vi "Page - Ports.vi"(8 "error in (no error)":errorcluster, 11 "Node Ptr":T3 format="%.0x") -> (0 "error out":errorcluster)   [LabVIEW 2020, in "SLSC-12201 DIO System Explorer.lvlib"]
uses:
  SLSC-12201 DIO System Explorer.lvlib
  <vilib>/NI VeriStand/Custom Device API/Custom Device API.lvlib
  <vilib>/NI VeriStand/Custom Device API/Custom Device Item Ref.ctl
  <vilib>/Utility/miscctls.llb/LVRowAndColumnTypeDef.ctl
  Direction Control.ctl
panel:
  in  "Apply":bool
  in  "Port Type":T1 items=["Input", "Output Source", "Output Sink", "Output Push-Pull"]
  out "Cell Position":T2
  in  "Type":u16(ring) items=["Input", "Output Source", "Output Sink", "Output Pull-up"]
  out "Multicolumn Listbox":i32(listbox)=4
  in  "Disable Port":bool
  in  "Enable Port":bool
  in  "SHDocVw.IWebBrowser2":refnum<k7>(container)
  in  "Header":cluster{"Section Name":string}={"Section Name"="Custom Device Item Settings"}
  in  "Description":string
  out "Name":string
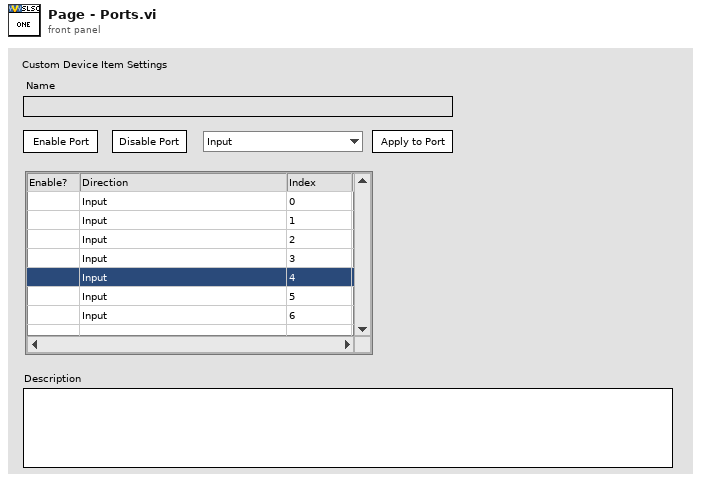
[diagram p1: front panel]
types:
  T1 = typedef "SLSC-12201 DIO System Explorer.lvlib/Direction Control.ctl" = u16
  T2 = typedef "LVRowAndColumnTypeDef.ctl" = cluster{"Row":i32, "Column":i32}
  T3 = typedef "Custom Device API.lvlib/Custom Device Item Ref.ctl" = u64
  T4 = typedef "Custom Device API.lvlib/Custom Device Item Info.ctl" = cluster{"Name":string, "Is Channel":bool, "GUID":string, "Is Waveform":bool}
  T5 = typedef "Custom Device API.lvlib/Custom Device Channel.ctl" = cluster{"Type":T6, "Units":string, "Default Value":dbl, "Faultable":bool, "Scalable":bool}
  T6 = typedef "Custom Device API.lvlib/Custom Device Channel Type.ctl" = enum16{"Input", "Output"}
  T7 = cluster{"Channel Name":string, "SLSC Name":string, "Channel":T5, "Enum Names":string[], "Enum Values":i32[]}[]
  T8 = typedef "Custom Device API.lvlib/Custom Device Commands.ctl" = enum16{"Default", "Item renamed", "Shutdown", "Dynamic button pressed"}
  T9 = typedef "LVPoint32TypeDef.ctl" = cluster{"Horizontal":i32, "Vertical":i32}
  T10 = typedef "LVPositionTypeDef.ctl" = cluster{"Left":i32, "Top":i32}
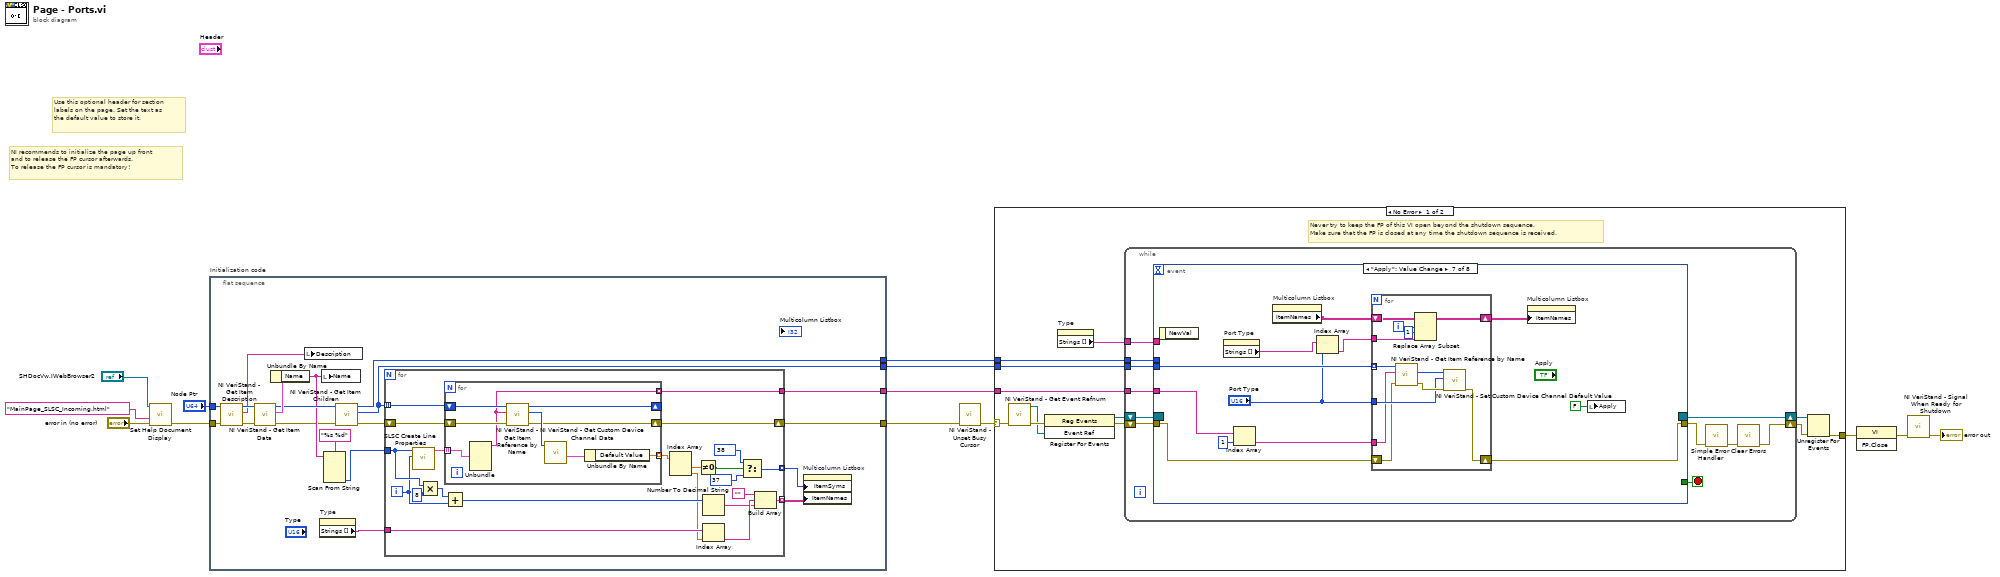
[diagram p0: block diagram]
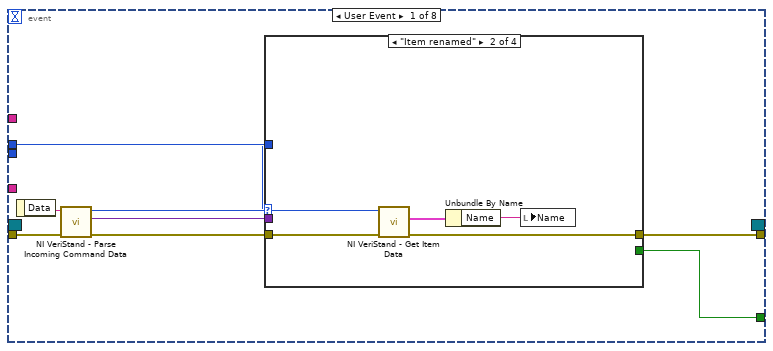
[diagram p2: hidden frame]
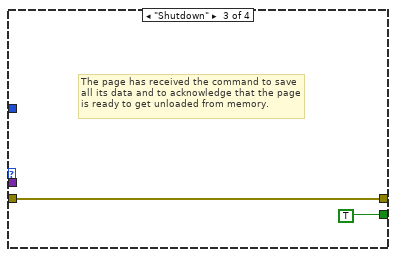
[diagram p4: hidden frame]
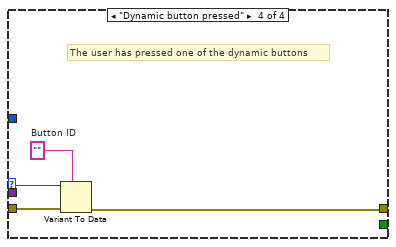
[diagram p5: hidden frame]
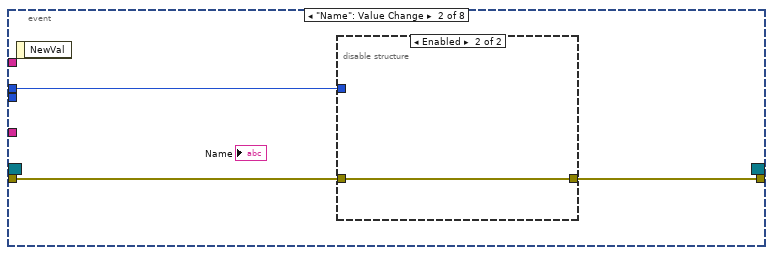
[diagram p6: hidden frame]
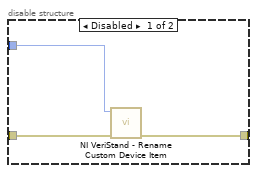
[diagram p7: hidden frame]
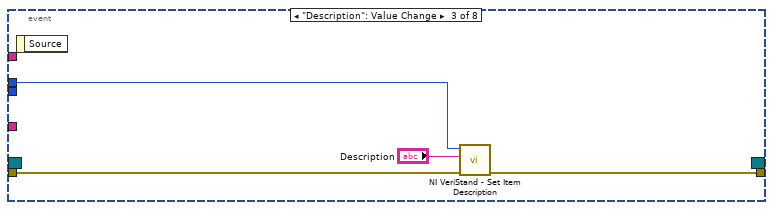
[diagram p8: hidden frame]
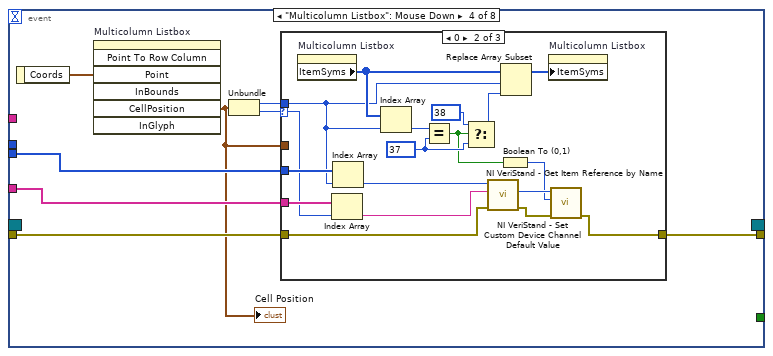
[diagram p9: hidden frame]
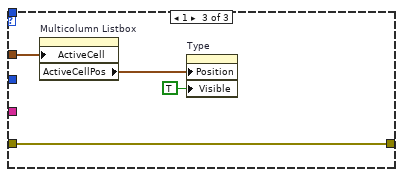
[diagram p11: hidden frame]
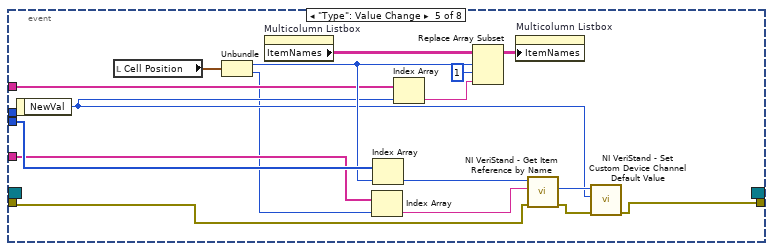
[diagram p12: hidden frame]
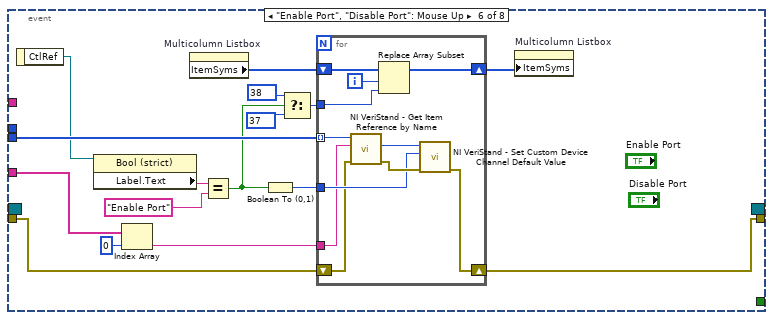
[diagram p13: hidden frame]
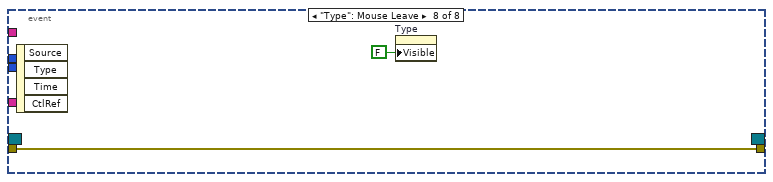
[diagram p14: hidden frame]
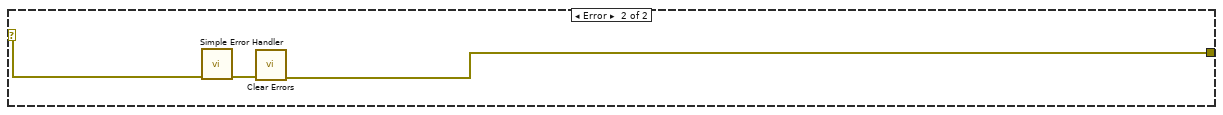
[diagram p15: hidden frame]
diagram:
  # "Use this optional header for section labels on the page. Set the text as the default value to store it."
  # "NI recommends to initialize the page up front\nand to release the FP cursor afterwards.\nTo release the FP cursor is mandatory!"
  n1 = call "Set Help Document Display.vi"("error in (no error)"="error in (no error)", "HTML File to Load"="MainPage_SLSC_Incoming.html" ("HTML File"), "SHDocVw.IWebBrowser2"="SHDocVw.IWebBrowser2") -> ("error out"=w3:errorcluster)  [unwired: 8 in]
  n2 = flat-sequence "Initialization code" {
    tunnel: w3 -> [w31]
    tunnel: "Node Ptr" -> [w30]
    tunnel: [w26] -> w9
    tunnel: [w24] -> w7
    tunnel: [w20] -> w2
    tunnel: [w19] -> w1
    frame #0 {
      n3 = call <vilib>:"NI VeriStand - Get Item Description.vi"("error in (no error)"=w31, "Item Ref in"=w30) -> ("error out"=w28:errorcluster, "Description"=w29:string, "Item Ref out"=w32:T3)  [unwired: 7 out]
      n4 = call <vilib>:"NI VeriStand - Get Item Data.vi"("error in (no error)"=w28, "Item Ref in"=w32) -> ("error out"=w18:errorcluster, "Item Info"=w27:T4, "Item Ref out"=w25:T3)  [unwired: 7 out]
      n5 = Unbundle By Name(w27) -> ("Name"=w22:string)
      n6 = local write "Description"(w29) -> ()
      n7 = property on="Type" class="Ring (strict)"() -> ("Strings []"=w16:string[])  [unwired: 2 in, 2 out]
      n8 = local write "Name"(w22) -> ()
      n9 = Scan From String(format string="%s %d", input string=w22) -> (output 2=w21:i32)  [unwired: 5 in, 3 out]
      n10 = call <vilib>:"NI VeriStand - Get Item Children.vi"("error in (no error)"=w18, "Item Ref in"=w25) -> ("error out"=w17:errorcluster, "Child Refs"=w20:T3[], "Item Ref out"=w24:T3)  [unwired: 6 in, 1 out]
      n11 = for {
        shift-right: [w53] -> w26
        shift-left: w17 -> [w54]
        tunnel: w20 -> [w50] mode=indexing
        tunnel: w21 -> [w47]
        tunnel: [w48] -> w19
        tunnel: w16 -> [w42]
        tunnel: [w37] -> w15 mode=indexing
        tunnel: [w33] -> w14 mode=indexing
        i -> [w44]
        n12 = call "SLSC Create Line Properties.vi"("Line Number"=w44, "Port Number"=w47) -> ("Outgoing configuration"=w52:T7)  [unwired: 9 in]
        n13 = Multiply(x=w47, y=8) -> (x*y=w45:i32)
        n14 = for {
          shift-right: [w60] -> w53
          shift-left: w54 -> [w61]
          shift-right: [w58] -> _
          shift-left: w50 -> [w59]
          tunnel: w52 -> [w57] mode=indexing
          tunnel: [w56] -> w51 mode=indexing
          tunnel: [w55] -> w48 mode=indexing
          n15 = Unbundle(w57) -> ("Channel Name"=w55:string)  [unwired: 4 out]
          n16 = call <vilib>:"NI VeriStand - Get Item Reference by Name.vi"("error in (no error)"=w61, "Item Name"=w55, "Parent Ref in"=w59) -> ("error out"=w60:errorcluster, "Item Ref"=w63:T3, "Parent Ref out"=w58:T3)  [unwired: 5 in, 1 out]
          n17 = call <vilib>:"NI VeriStand - Get Custom Device Channel Data.vi"("Channel Ref in"=w63) -> ("Channel"=w62:T5)  [unwired: 5 in, 5 out]
          n18 = Unbundle By Name(w62) -> ("Default Value"=w56:dbl)
        }
        n19 = Add(x=w45, y=w44) -> (x+y=w43:i32)
        n20 = Index Array(array=w51) -> (element #1=w49:dbl, element #2=w41:dbl)  [unwired: 2 in]
        n21 = Not Equal To 0?(x=w49) -> (x != 0?=w38:bool)
        n22 = Number To Decimal String(number=w43) -> (decimal integer string=w34:string)  [unwired: 1 in]
        n23 = Index Array(array=w42, index=w41) -> (element=w35:string)
        n24 = Select(t=38, s=w38, f=37) -> (s? t:f=w37:i32)
        n25 = Build Array("", w35, w34) -> (w33:string[])
      }
      n26 = property on="Multicolumn Listbox" class="MCListbox (strict)"("ItemSyms"=w15, "ItemNames"=w14) -> ()  [unwired: 2 in, 2 out]
    }
  }
  n27 = call <vilib>:"NI VeriStand - Unset Busy Cursor.vi"("error in (no error)"=w9) -> ("error out"=w8:errorcluster)  [unwired: 10 out]
  n28 = case shown="No Error" w8 {
    selector: w8 -> [w67 w221]
    tunnel: [w72 w219] -> w13
    tunnel: w7 -> [w68 _]
    tunnel: w2 -> [w66 _]
    tunnel: w1 -> [w65 _]
    frame No Error {
      # "Never try to keep the FP of this VI open beyond the shutdown sequence.\nMake sure that the FP is closed at any time the shutdown sequence is received."
      n29 = call <vilib>:"NI VeriStand - Get Event Refnum.vi"("error in (no error)"=w67) -> ("error out"=w75:errorcluster, "Event Ref"=w71:refnum<user-event>)  [unwired: 9 out]
      n30 = register-events(error in=w75, w71) -> (reference out=w69:refnum<event-registration>, error out=w70:errorcluster)  [unwired: 1 in]
      n31 = property on="Type" class="Ring (strict)"() -> ("Strings []"=w64:string[])  [unwired: 2 in, 2 out]
      n32 = while {
        tunnel: w68 -> [w82]
        shift-right: [w79] -> w73
        shift-left: w70 -> [w85]
        shift-right: [w86] -> w74
        shift-left: w69 -> [w84]
        tunnel: w66 -> [w78]
        tunnel: w65 -> [w77]
        tunnel: w64 -> [w76]
        stop <- w83 stop-if-true
        n33 = event shown="[6] \"Apply\": Value Change" {
          selector: w84 -> [_ _ _ _ _ _ _ _]
          dyn-events: [_ _ _ _ _ _ _ _] -> w86
          timeout: _ -> [_ _ _ _ _ _ _ _]
          tunnel: w85 -> [w94 w109 w116 w120 w152 w171 w200 w218]
          tunnel: [w90 _ _ _ _ _ _ _] -> w83
          tunnel: [w89 w108 w115 w119 w150 w170 w199 w218] -> w81
          tunnel: w82 -> [w88 w107 w117 _ _ _ _ _]
          tunnel: w78 -> [_ _ _ w122 w156 w181 w204 _]
          tunnel: w77 -> [_ _ _ w121 w155 w174 w203 _]
          tunnel: w76 -> [_ _ _ _ w151 _ _ _]
          event User Event {
            n34 = event-data() -> ("Data"=w93:string)  [unwired: 1 out]
            n35 = call <vilib>:"NI VeriStand - Parse Incoming Command Data.vi"("error in (no error)"=w94, "Incoming data"=w93) -> ("error out"=w92:errorcluster, "Outgoing data"=w87:variant, "Action"=w91:T8)  [unwired: 7 out]
            n36 = case shown="\"Item renamed\"" w91 {
              tunnel: w92 -> [w95 w100 w101 w106]
              tunnel: [_ _ TRUE _] -> w90
              tunnel: [w95 w97 w101 w103] -> w89
              tunnel: w88 -> [_ w99 _ _]
              tunnel: w87 -> [_ _ _ w105]
              frame "Default", Default {
              }
              frame "Item renamed" {
                n37 = call <vilib>:"NI VeriStand - Get Item Data.vi"("error in (no error)"=w100, "Item Ref in"=w99) -> ("error out"=w97:errorcluster, "Item Info"=w98:T4)  [unwired: 8 out]
                n38 = Unbundle By Name(w98) -> ("Name"=w96:string)
                n39 = local write "Name"(w96) -> ()
              }
              frame "Shutdown" {
                # "The page has received the command to save all its data and to acknowledge that the page is ready to get unloaded from memory."
              }
              frame "Dynamic button pressed" {
                w104 = ""  # Button ID
                # "The user has pressed one of the dynamic buttons"
                n40 = Variant To Data(error in=w106, type=w104, Variant=w105) -> (error out=w103:errorcluster)  [unwired: 1 out]
              }
            }
          }
          event "Name": Value Change {
            n41 = event-data() -> ()  [unwired: 2 out]
            n42 = disable-structure shown="Enabled" {
              disable-tunnel: w109 -> [w112 w113]
              disable-tunnel: [w111 w113] -> w108
              disable-tunnel: w107 -> [w110 _]
              frame Disabled {
                n43 = call <vilib>:"NI VeriStand - Rename Custom Device Item.vi"("error in (no error)"=w112, "Item Ref in"=w110) -> ("error out"=w111:errorcluster)  [unwired: 2 in, 7 out]
              }
              frame Enabled {
              }
            }
          }
          event "Description": Value Change {
            n44 = event-data() -> ()  [unwired: 2 out]
            n45 = call <vilib>:"NI VeriStand - Set Item Description.vi"("error in (no error)"=w116, "Description"="Description", "Item Ref in"=w117) -> ("error out"=w115:errorcluster)  [unwired: 8 out]
          }
          event "Multicolumn Listbox": Mouse Down {
            n46 = event-data() -> ("Coords"=w125:T9)  [unwired: 1 out]
            n47 = invoke on="Multicolumn Listbox" class="MCListbox (strict)" method="Point To Row Column"("Point"=w125) -> ("CellPosition"=w118:T2)  [unwired: 6 in, 6 out]
            "Cell Position" <- w118
            n48 = Unbundle(w118) -> ("Row"=w123:i32, "Column"=w124:i32)
            n49 = case shown="0" w124 {
              selector: w124 -> [_ w127 _]
              tunnel: w123 -> [_ w133 _]
              tunnel: w122 -> [_ w138 _]
              tunnel: w121 -> [_ w134 _]
              tunnel: w120 -> [w126 w129 w145]
              tunnel: [w126 w128 w145] -> w119
              tunnel: w118 -> [_ _ w148]
              frame 2, Default {
              }
              frame 0 {
                w143 = 37
                n50 = property on="Multicolumn Listbox" class="MCListbox (strict)"() -> ("ItemSyms"=w140:i32[])  [unwired: 2 in, 2 out]
                n51 = Index Array(array=w134, index=w127) -> (element=w132:string)
                n52 = Index Array(array=w138, index=w133) -> (element=w135:T3)
                n53 = Index Array(array=w140, index=w133) -> (element=w142:i32)
                n54 = Equal?(x=w142, y=w143) -> (x = y?=w131:bool)
                n55 = Select(t=38, s=w131, f=w143) -> (s? t:f=w141:i32)
                n56 = call <vilib>:"NI VeriStand - Get Item Reference by Name.vi"("error in (no error)"=w129, "Item Name"=w132, "Parent Ref in"=w135) -> ("error out"=w137:errorcluster, "Item Ref"=w136:T3)  [unwired: 5 in, 2 out]
                n57 = Boolean To (0,1)(Boolean=w131) -> (0, 1=w130:i16)
                n58 = Replace Array Subset(array=w140, new element=w141, index=w133) -> (w139:i32[])
                n59 = property on="Multicolumn Listbox" class="MCListbox (strict)"("ItemSyms"=w139) -> ()  [unwired: 2 in, 2 out]
                n60 = call <vilib>:"NI VeriStand - Set Custom Device Channel Default Value.vi"("error in (no error)"=w137, "Default Value"=w130, "Channel Ref in"=w136) -> ("error out"=w128:errorcluster)  [unwired: 7 in, 1 out]
              }
              frame 1 {
                n61 = property on="Multicolumn Listbox" class="MCListbox (strict)"("ActiveCell"=w148) -> ("ActiveCellPos"=w147:T10)  [unwired: 2 in, 2 out]
                n62 = property on="Type" class="Ring (strict)"("Position"=w147, "Visible"=TRUE) -> ()  [unwired: 2 in, 2 out]
              }
            }
          }
          event "Type": Value Change {
            n63 = event-data() -> ("NewVal"=w153:u16)  [unwired: 1 out]
            n64 = local read "Cell Position"() -> (w162:T2)
            n65 = Unbundle(w162) -> ("Row"=w154:i32, "Column"=w149:i32)
            n66 = property on="Multicolumn Listbox" class="MCListbox (strict)"() -> ("ItemNames"=w165:string[][])  [unwired: 2 in, 2 out]
            n67 = Index Array(array=w155, index=w149) -> (element=w157:string)
            n68 = Index Array(array=w156, index=w154) -> (element=w158:T3)
            n69 = Index Array(array=w151, index=w153) -> (element=w161:string)
            n70 = Replace Array Subset(array=w165, new element=w161, index (row)=w154, index (col)=1 ("disabled index (col)")) -> (w164:string[][])
            n71 = property on="Multicolumn Listbox" class="MCListbox (strict)"("ItemNames"=w164) -> ()  [unwired: 2 in, 2 out]
            n72 = call <vilib>:"NI VeriStand - Get Item Reference by Name.vi"("error in (no error)"=w152, "Item Name"=w157, "Parent Ref in"=w158) -> ("error out"=w160:errorcluster, "Item Ref"=w159:T3)  [unwired: 5 in, 2 out]
            n73 = call <vilib>:"NI VeriStand - Set Custom Device Channel Default Value.vi"("error in (no error)"=w160, "Default Value"=w153, "Channel Ref in"=w159) -> ("error out"=w150:errorcluster)  [unwired: 7 in, 1 out]
          }
          event "Enable Port", "Disable Port": Mouse Up {
            n74 = event-data() -> ("CtlRef"=w178:refnum<vi>)  [unwired: 1 out]
            n75 = property class="Bool (strict)"(reference=w178) -> ("Label.Text"=w177:string)  [unwired: 1 in, 2 out]
            n76 = Index Array(array=w174, index=0) -> (element=w172:string)
            n77 = property on="Multicolumn Listbox" class="MCListbox (strict)"() -> ("ItemSyms"=w180:i32[])  [unwired: 2 in, 2 out]
            n78 = Equal?(x=w177, y="Enable Port") -> (x = y?=w169:bool)
            n79 = Boolean To (0,1)(Boolean=w169) -> (0, 1=w175:i16)
            n80 = Select(t=38, s=w169, f=37) -> (s? t:f=w166:i32)
            n81 = for {
              tunnel: w181 -> [w190] mode=indexing
              shift-right: [w187] -> w179
              shift-left: w180 -> [w188]
              tunnel: w175 -> [w186]
              tunnel: w172 -> [w185]
              shift-right: [w183] -> w170
              shift-left: w171 -> [w184]
              tunnel: w166 -> [w182]
              i -> [w189]
              n82 = call <vilib>:"NI VeriStand - Get Item Reference by Name.vi"("error in (no error)"=w184, "Item Name"=w185, "Parent Ref in"=w190) -> ("error out"=w192:errorcluster, "Item Ref"=w191:T3)  [unwired: 5 in, 2 out]
              n83 = Replace Array Subset(array=w188, new element=w182, index=w189) -> (w187:i32[])
              n84 = call <vilib>:"NI VeriStand - Set Custom Device Channel Default Value.vi"("error in (no error)"=w192, "Default Value"=w186, "Channel Ref in"=w191) -> ("error out"=w183:errorcluster)  [unwired: 7 in, 1 out]
            }
            n85 = property on="Multicolumn Listbox" class="MCListbox (strict)"("ItemSyms"=w179) -> ()  [unwired: 2 in, 2 out]
          }
          event "Apply": Value Change {
            n86 = event-data() -> ()  [unwired: 2 out]
            n87 = property on="Port Type" class="Ring (strict)"() -> ("Strings []"=w196:string[])  [unwired: 2 in, 2 out]
            n88 = Index Array(array=w203, index=1) -> (element=w201:string)
            n89 = property on="Multicolumn Listbox" class="MCListbox (strict)"() -> ("ItemNames"=w198:string[][])  [unwired: 2 in, 2 out]
            n90 = Index Array(array=w196, index="Port Type") -> (element=w194:string)
            n91 = for {
              tunnel: w204 -> [w214] mode=indexing
              shift-right: [w211] -> w197
              shift-left: w198 -> [w212]
              tunnel: "Port Type" -> [w210]
              tunnel: w201 -> [w209]
              shift-right: [w207] -> w199
              shift-left: w200 -> [w208]
              tunnel: w194 -> [w205]
              i -> [w213]
              n92 = call <vilib>:"NI VeriStand - Get Item Reference by Name.vi"("error in (no error)"=w208, "Item Name"=w209, "Parent Ref in"=w214) -> ("error out"=w216:errorcluster, "Item Ref"=w215:T3)  [unwired: 5 in, 2 out]
              n93 = Replace Array Subset(array=w212, new element=w205, index (row)=w213, index (col)=1 ("disabled index (col)")) -> (w211:string[][])
              n94 = call <vilib>:"NI VeriStand - Set Custom Device Channel Default Value.vi"("error in (no error)"=w216, "Default Value"=w210, "Channel Ref in"=w215) -> ("error out"=w207:errorcluster)  [unwired: 7 in, 1 out]
            }
            n95 = property on="Multicolumn Listbox" class="MCListbox (strict)"("ItemNames"=w197) -> ()  [unwired: 2 in, 2 out]
            n96 = local write "Apply"(FALSE ("Apply")) -> ()
          }
          event "Type": Mouse Leave {
            n97 = event-data() -> ()  [unwired: 5 out]
            n98 = property on="Type" class="Ring (strict)"("Visible"=FALSE) -> ()  [unwired: 2 in, 2 out]
          }
        }
        n99 = call <vilib>:"Simple Error Handler.vi"("error in (no error)"=w81) -> ("error out"=w80:errorcluster)  [unwired: 1 in, 7 out]
        n100 = call <vilib>:"Clear Errors.vi"("error in (no error)"=w80) -> ("error out"=w79:errorcluster)  [unwired: 1 in, 5 out]
      }
      n101 = Unregister For Events(event registration refnum=w74, error in=w73) -> (error out=w72:errorcluster)
    }
    frame Error {
      n102 = call <vilib>:"Simple Error Handler.vi"("error in (no error)"=w221) -> ("error out"=w220:errorcluster)  [unwired: 1 in, 7 out]
      n103 = call <vilib>:"Clear Errors.vi"("error in (no error)"=w220) -> ("error out"=w219:errorcluster)  [unwired: 1 in, 5 out]
    }
  }
  n104 = invoke class="VI" method="FP.Close"(error in=w13) -> (error out=w12:errorcluster)  [unwired: 2 in, 2 out]
  n105 = call <vilib>:"NI VeriStand - Signal When Ready for Shutdown.vi"("error in (no error)"=w12) -> ("error out"=→"error out":errorcluster)  [unwired: 10 out]
